vi "CMD_Drive.vi"(1 "Line":string) -> (0 "Done":bool)   [LabVIEW 2015]
uses:
  <vilib>/Rock Robotics/WPI/RobotDrive/WPI_RobotDriveGetSetRefNum.vi
panel:
  out "Error":string
  in  "Parameters":i32[](array[numeric])=[1, 1, 2, 2]
  in  "Subcommands":string[](array[string])=["at", "for", "speed", "turn"]
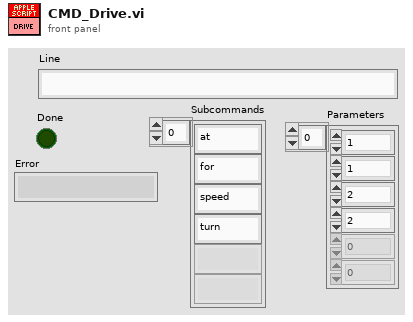
[diagram p1: front panel]
types:
  T1 = typedef "WPI_RobotDriveDevRef.ctl" = cluster{"DevStatus":errorcluster, "Motors[]":T2[], "Square Inputs":bool, "Max Output":dbl}
  T2 = typedef "WPI_MotorControlDeviceRef.ctl" = cluster{"DeviceStatus":errorcluster, "Type":enum16{"PWM", "CAN"}, "PWM":cluster{"Digital Module":T3, "PWM Channel":T4, "DeadBand":T5}, "CAN":cluster{"Device Number":u8, "Control Mode":T6, "Semaphore":T7, "Max Vout":dbl}, "Invert":bool, "TransformRef":T8, "InvTransformRef":T8}
  T3 = typedef "FPGA_TypedefDigitalModule.ctl" = enum16{"Digital Module 1", "Digital Module 2"}
  T4 = typedef "FPGA_DIOPWMChannel.ctl" = enum8{"PWM 1", "PWM 2", "PWM 3", "PWM 4", "PWM 5", "PWM 6", "PWM 7", "PWM 8", "PWM 9", "PWM 10", "Invalid"}
  T5 = typedef "WPI_PWMDeadband.ctl" = cluster{"Name":string, "maxPositivePwm":i32, "minPositivePwm":i32, "centerPwm":i32, "maxNegativePwm":i32, "minNegativePwm":i32, "angularRange":u16}
  T6 = typedef "WPI_CANJaguar_ControlMode.ctl" = enum8{"Percent VBus", "Current", "Speed", "Position", "Voltage"}
  T7 = typedef "Semaphore RefNum" = refnum<k1>
  T8 = typedef "WPI_PWMTransform_ConPane.ctl" = refnum<vi>
  T9 = typedef "WPI_GyroDevRef.ctl" = cluster{"DevStatus":errorcluster, "Analog Module":T10, "Analog Channel":T11, "Offset":dbl, "Gain (VoltsPerDegree/Second)":dbl}
  T10 = typedef "FPGA_TypedefAnalogModule.ctl" = enum16{"Analog Module 1", "Analog Module 2"}
  T11 = typedef "FPGA_AIChannel.ctl" = enum8{"AI 1", "AI 2", "AI 3", "AI 4", "AI 5", "AI 6", "AI 7", "AI 8", "Invalid"}
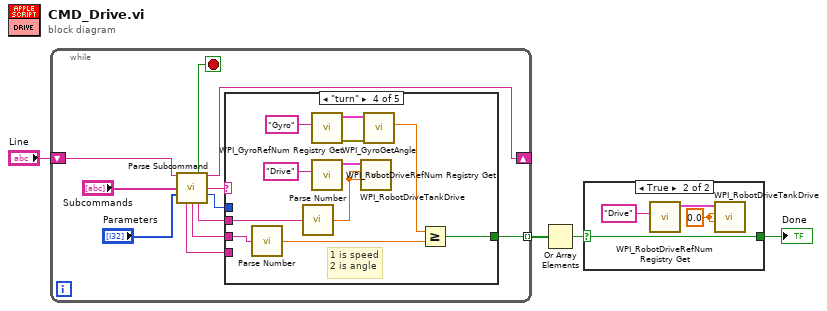
[diagram p0: block diagram]
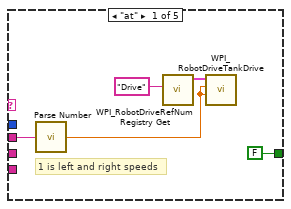
[diagram p3: hidden frame]
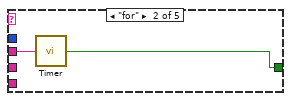
[diagram p4: hidden frame]
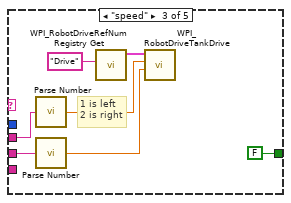
[diagram p5: hidden frame]
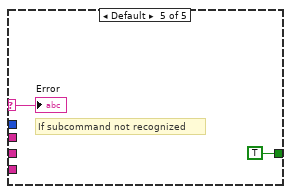
[diagram p6: hidden frame]
diagram:
  n1 = while {
    shift-right: [w12] -> _
    shift-left: "Line" -> [w15]
    tunnel: [w5] -> w3 mode=indexing
    stop <- w11 stop-if-true
    n2 = call "Parse Subcommand.vi"("Text In"=w15, "Subcommands"="Subcommands", "Parameters"="Parameters") -> ("Done"=w11:bool, "Text Out"=w12:string, "Subcommand"=w10:string, "# of Parameters"=w9:i32, "Parameter 3"=w6:string, "Parameter 2"=w7:string, "Parameter 1"=w8:string)  [unwired: 6 in]
    n3 = case shown="\"turn\"" w10 {
      selector: w10 -> [_ _ _ _ w41]
      tunnel: w9 -> [_ _ _ _ _]
      tunnel: w8 -> [w18 w22 w27 w38 _]
      tunnel: w7 -> [_ _ w26 w37 _]
      tunnel: w6 -> [_ _ _ _ _]
      tunnel: [FALSE ("Done") w21 FALSE ("Done") w30 TRUE] -> w5
      frame "at" {
        # "1 is left and right speeds"
        n4 = call "Parse Number.vi"("String"=w18) -> ("Number"=w17:dbl)
        n5 = call <vilib>:"WPI_RobotDriveRefNum Registry Get.vi"("refnum name"="Drive") -> ("RobotDriveDevRef"=w19:T1)  [unwired: 9 in, 1 out]
        n6 = call <vilib>:"WPI_RobotDriveTankDrive.vi"("Right axis value"=w17, "Left axis value"=w17, "RobotDriveDevRef"=w19) -> ()  [unwired: 6 in, 3 out]
      }
      frame "for" {
        n7 = call "Timer.vi"("Seconds (string)"=w22) -> ("Done"=w21:bool)
      }
      frame "speed" {
        # "1 is left\n2 is right"
        n8 = call "Parse Number.vi"("String"=w27) -> ("Number"=w24:dbl)
        n9 = call "Parse Number.vi"("String"=w26) -> ("Number"=w25:dbl)
        n10 = call <vilib>:"WPI_RobotDriveRefNum Registry Get.vi"("refnum name"="Drive") -> ("RobotDriveDevRef"=w28:T1)  [unwired: 9 in, 1 out]
        n11 = call <vilib>:"WPI_RobotDriveTankDrive.vi"("Right axis value"=w25, "Left axis value"=w24, "RobotDriveDevRef"=w28) -> ()  [unwired: 6 in, 3 out]
      }
      frame "turn" {
        # "1 is speed\n2 is angle"
        n12 = call "Parse Number.vi"("String"=w37) -> ("Number"=w31:dbl)
        n13 = call "Parse Number.vi"("String"=w38) -> ("Number"=w33:dbl)
        n14 = call <vilib>:"WPI_GyroRefNum Registry Get.vi"("refnum name"="Gyro") -> ("error out"=w36:errorcluster, "GyroDevRef"=w35:T9)  [unwired: 9 in]
        n15 = call <vilib>:"WPI_RobotDriveRefNum Registry Get.vi"("refnum name"="Drive") -> ("RobotDriveDevRef"=w39:T1)  [unwired: 9 in, 1 out]
        n16 = call <vilib>:"WPI_RobotDriveTankDrive.vi"("Right axis value"=w33, "Left axis value"=w33, "RobotDriveDevRef"=w39) -> ()  [unwired: 6 in, 3 out]
        n17 = call <vilib>:"WPI_GyroGetAngle.vi"("error in (no error)"=w36, "GyroDevRef"=w35) -> ("Angle"=w32:dbl)  [unwired: 6 in, 3 out]
        n18 = Greater Or Equal?(x=w32, y=w31) -> (x >= y?=w30:bool)
      }
      frame Default {
        # "If subcommand not recognized"
        "Error" <- w41
      }
    }
  }
  n19 = Or Array Elements(Boolean array=w3) -> (logical OR=w2:bool)
  n20 = case shown="True" w2 {
    selector: w2 -> [w43 w44]
    tunnel: [w43 w44] -> w1
    frame False {
    }
    frame True {
      w45 = 0.0 ("Left axis value")
      n21 = call <vilib>:"WPI_RobotDriveRefNum Registry Get.vi"("refnum name"="Drive") -> ("RobotDriveDevRef"=w46:T1)  [unwired: 9 in, 1 out]
      n22 = call <vilib>:"WPI_RobotDriveTankDrive.vi"("Right axis value"=w45, "Left axis value"=w45, "RobotDriveDevRef"=w46) -> ()  [unwired: 6 in, 3 out]
    }
  }
  "Done" <- w1
